vi "Start CONV.vi"(1 "Orig Config":u8[](array[numeric])) -> (0 "New Config":u8[](array[numeric]))   [LabVIEW 2021]
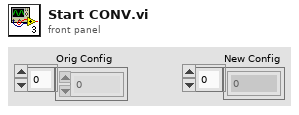
[diagram p1: front panel]
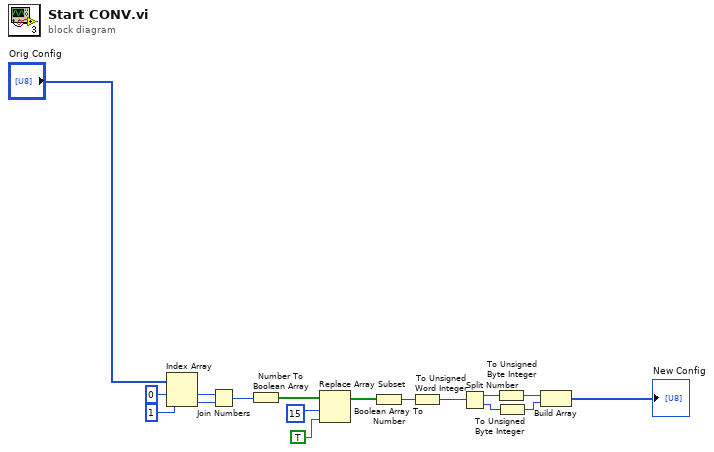
[diagram p0: block diagram]
diagram:
  n1 = Index Array(array="Orig Config", index #1=0 ("index"), index #2=1 ("index")) -> (element #1=w3:u8, element #2=w4:u8)
  n2 = Join Numbers(hi=w3, lo=w4) -> ((hi.lo)=w5:u16)
  n3 = Number To Boolean Array(number=w5) -> (Boolean array=w7:bool[])
  n4 = Replace Array Subset(array=w7, new element=TRUE ("new element/subarray"), index=15) -> (w15:bool[])
  n5 = Boolean Array To Number(Boolean array=w15) -> (number=w13:u32)
  n6 = To Unsigned Word Integer(number=w13) -> (unsigned 16bit integer=w14:u16)
  n7 = Split Number(x=w14) -> (hi(x)=w9:u8, lo(x)=w11:u8)
  n8 = To Unsigned Byte Integer(number=w9) -> (unsigned 8bit integer=w10:u8)
  n9 = To Unsigned Byte Integer(number=w11) -> (unsigned 8bit integer=w12:u8)
  n10 = Build Array(w10, w12) -> (→"New Config":u8[])
